vi "DAQmx.Start AI.vi"(6 "error in (no error)":errorcluster, 9 "DAQmx in":refnum<class "DAQmx.lvclass">) -> (0 "error out":errorcluster, 3 "DAQmx out":refnum<class "DAQmx.lvclass">)   [LabVIEW 2019, in "DAQmx.lvclass"]
uses:
  DAQmx.lvclass
  DAQmx.lvclass/DAQmx.ctl
  <vilib>/DAQmx/read.llb/DAQmx Read (Analog 1D Wfm NChan NSamp).vi
  <vilib>/DAQmx/miscellaneous.llb/DAQmx Fill In Error Info.vi
  <resource>/objmgr/daqmx.rc
panel:
  out "Devices":tag[](array[tag])
  out "data":waveform(dbl)[](array[waveform])
  out "Samples to read":i32[](array[numeric])
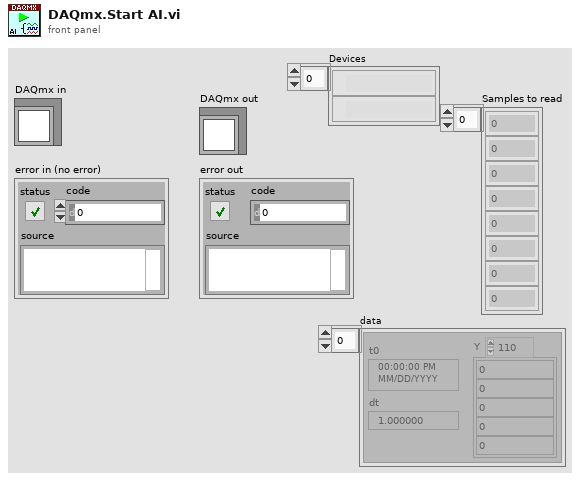
[diagram p1: front panel]
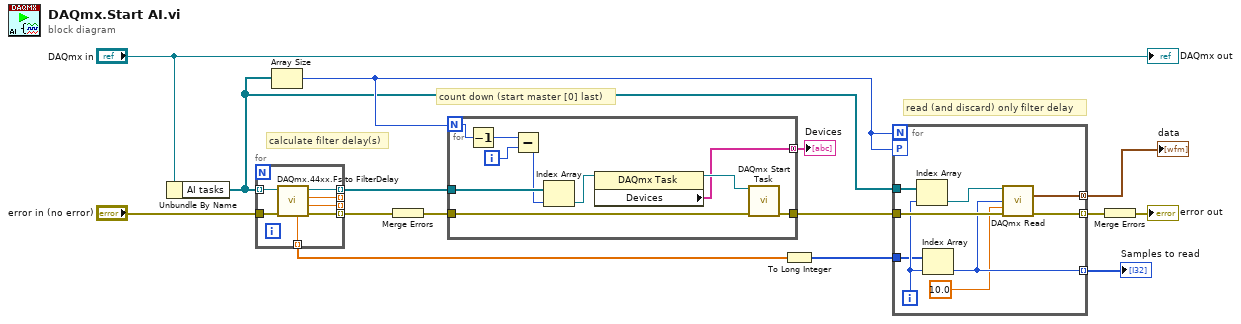
[diagram p0: block diagram]
diagram:
  # "read (and discard) only filter delay"
  # "calculate filter delay(s)"
  # "count down (start master [0] last)"
  n1 = Unbundle By Name("DAQmx in") -> ("AI tasks"=w6:refnum<k21>[])
  n2 = for {
    tunnel: w6 -> [w22] mode=indexing
    tunnel: [w21] -> w13 mode=indexing
    tunnel: [w20] -> _ mode=indexing
    tunnel: [w19] -> w11 mode=indexing
    tunnel: "error in (no error)" -> [w18]
    tunnel: [w17] -> _ mode=indexing
    tunnel: [w16] -> w5 mode=indexing
    n3 = call "DAQmx.44xx.Fs to FilterDelay.vi"("error in (no error)"=w18, "Refnum in"=w22) -> ("error out"=w19:errorcluster, "DAC Delay (samples)"=w17:dbl, "ADC Delay (samples)"=w20:dbl, "Refnum out"=w21:refnum<k21>, "Total Filter Delay (samples)"=w16:dbl)  [unwired: 5 in]
  }
  n4 = Array Size(array=w6) -> (size(s)=w7:i32)
  n5 = Merge Errors(w11) -> (w10:errorcluster)
  n6 = for {
    N: w7 -> [w28]
    tunnel: w10 -> [w32]
    tunnel: [w31] -> w9
    tunnel: w13 -> [w29]
    tunnel: [w23] -> w2 mode=concatenating
    i -> [w27]
    n7 = Decrement(x=w28) -> (x-1=w25:i32)
    n8 = Subtract(x=w25, y=w27) -> (x-y=w26:i32)
    n9 = Index Array(array=w29, index=w26) -> (element=w30:refnum<k21>)
    n10 = property class="DAQmx Task"(reference=w30) -> (reference out=w24:refnum<k21>, "Devices"=w23:tag[])  [unwired: 1 in, 1 out]
    n11 = call <vilib>:"DAQmx Start Task.vi"("task/channels in"=w24, "error in"=w32) -> ("error out"=w31:errorcluster)  [unwired: 12 in, 1 out]
  }
  "Devices" <- w2
  n12 = To Long Integer(number=w5) -> (32bit integer=w4:i32[])
  n13 = for {
    N: w7 -> [_]
    tunnel: w6 -> [w39]
    workers-P: w7 -> [_]
    tunnel: w9 -> [w41]
    tunnel: [w40] -> w8 mode=indexing
    tunnel: w4 -> [w36]
    tunnel: [w35] -> w3 mode=concatenating
    tunnel: [w34] -> w1 mode=indexing
    i -> [w38]
    n14 = Index Array(array=w39, index=w38) -> (element=w37:refnum<k21>)
    n15 = Index Array(array=w36, index=w38) -> (element=w34:i32)
    n16 = call-poly <vilib>:"DAQmx Read.vi"("task/channels in"=w37, "number of samples per channel"=w34, "timeout"=10.0, "error in"=w41) -> ("data"=w35:waveform(dbl)[], "error out"=w40:errorcluster)  [unwired: 9 in, 1 out]
  }
  "Samples to read" <- w1
  "data" <- w3
  n17 = Merge Errors(w8) -> (→"error out":errorcluster)
  "DAQmx out" <- "DAQmx in"
